vi "Set Session Property (DBL).vi"(0 "session in":refnum<k21>, 7 "property":refnum<k21>, 9 "property value":dbl, 11 "error in (no error)":errorcluster) -> (4 "session out":refnum<k21>, 15 "error out":errorcluster)   [LabVIEW 2020, in "SLSC.lvlib"]
uses:
  <vilib>/SLSC/SLSC.lvlib
  nislsclvapi.dll
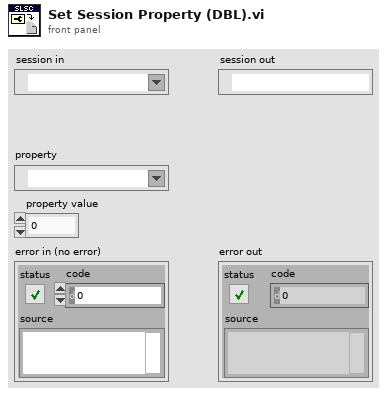
[diagram p1: front panel]
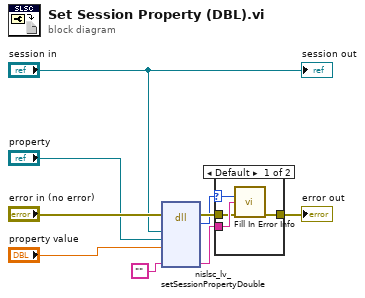
[diagram p0: block diagram]
diagram:
  n1 = dll-call lib="nislsclvapi.*" fn="nislsc_lv_setSessionPropertyDouble"(error in="error in (no error)", "session"="session in", "property"="property", "propertyValue"="property value", "extendedErrorInfo"="") -> (error out=w6:errorcluster, w5:i32, "extendedErrorInfo"=w7:string)  [unwired: 7 in, 1 out]
  n2 = case shown="Default" w5 {
    selector: w5 -> [w13 _]
    tunnel: w7 -> [w12 _]
    tunnel: w6 -> [w11 w14]
    tunnel: [w10 w14] -> w4
    frame Default {
      n3 = call <vilib>:"Fill In Error Info.vi"("status code"=w13, "extended error info"=w12, "error in"=w11) -> ("error out"=w10:errorcluster)  [unwired: 12 in]
    }
    frame 0 {
    }
  }
  "error out" <- w4
  "session out" <- "session in"
